vi "更新update.vi"() -> ()   [LabVIEW 2016, in "自动更新.lvlib"]
uses:
  <vilib>/FTP/NI_FTP.lvlib
panel:
  out "本地路径":path
  out "FTP链接结束":bool
  out "更新进度":u8(slide) scale=0.0..100.0
  # "更新update，请稍后！"
  # "s"
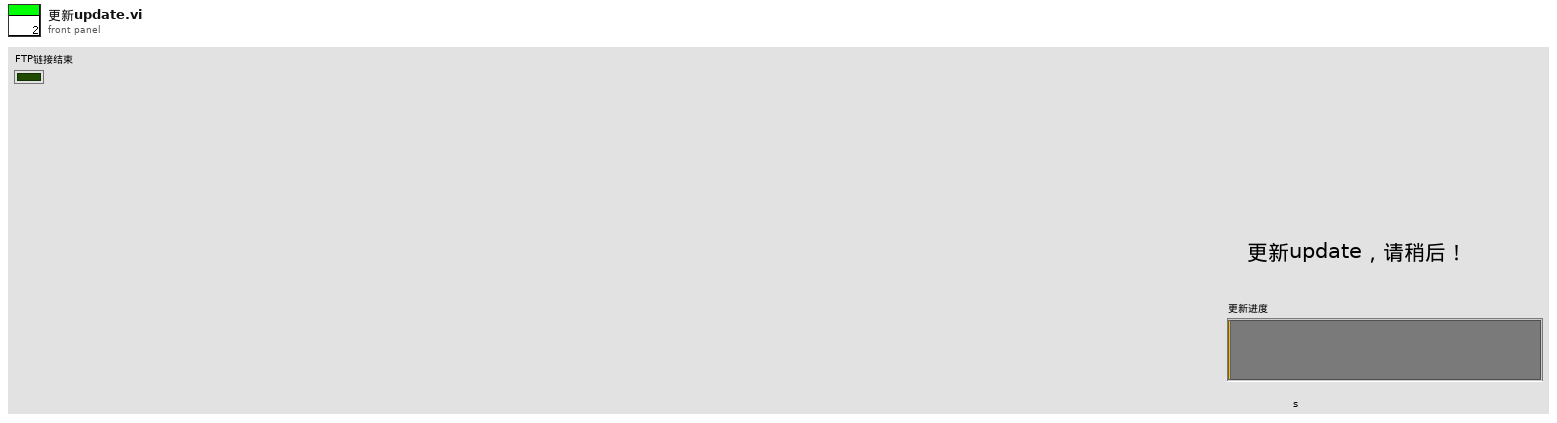
[diagram p1: front panel]
types:
  T1 = enum16{"get version information", "get success", "contact", "over"}
  T2 = cluster{"网络灯":bool, "接收中":bool, "已接收百分比":u8, "接收成功次数":dbl, "当前步骤":enum16{"init", "receivehead", "receivecontent", "receivesuccess", "over"}, "文件名":string, "error out":errorcluster}
  T3 = cluster{"remote path":string, "local path":path, "binary":bool}
  T4 = cluster{"主机":string, "用户":string, "密码":string, "远程路径":string, "下载文件名":string, "软件版本":string}
  T5 = typedef "NI_FTP.lvlib/FTP Session.ctl" = refnum<k5>
  T6 = typedef "NI_FTP.lvlib/FTP File Info.ctl" = cluster{"type":enum16{"unknown", "file", "dir", "link"}, "permissions":string, "owner":string, "group":string, "size":i32, "date":string, "name":string, "link name":string}
  T7 = cluster{"remote path":string, "local path":path, "binary":bool}[]
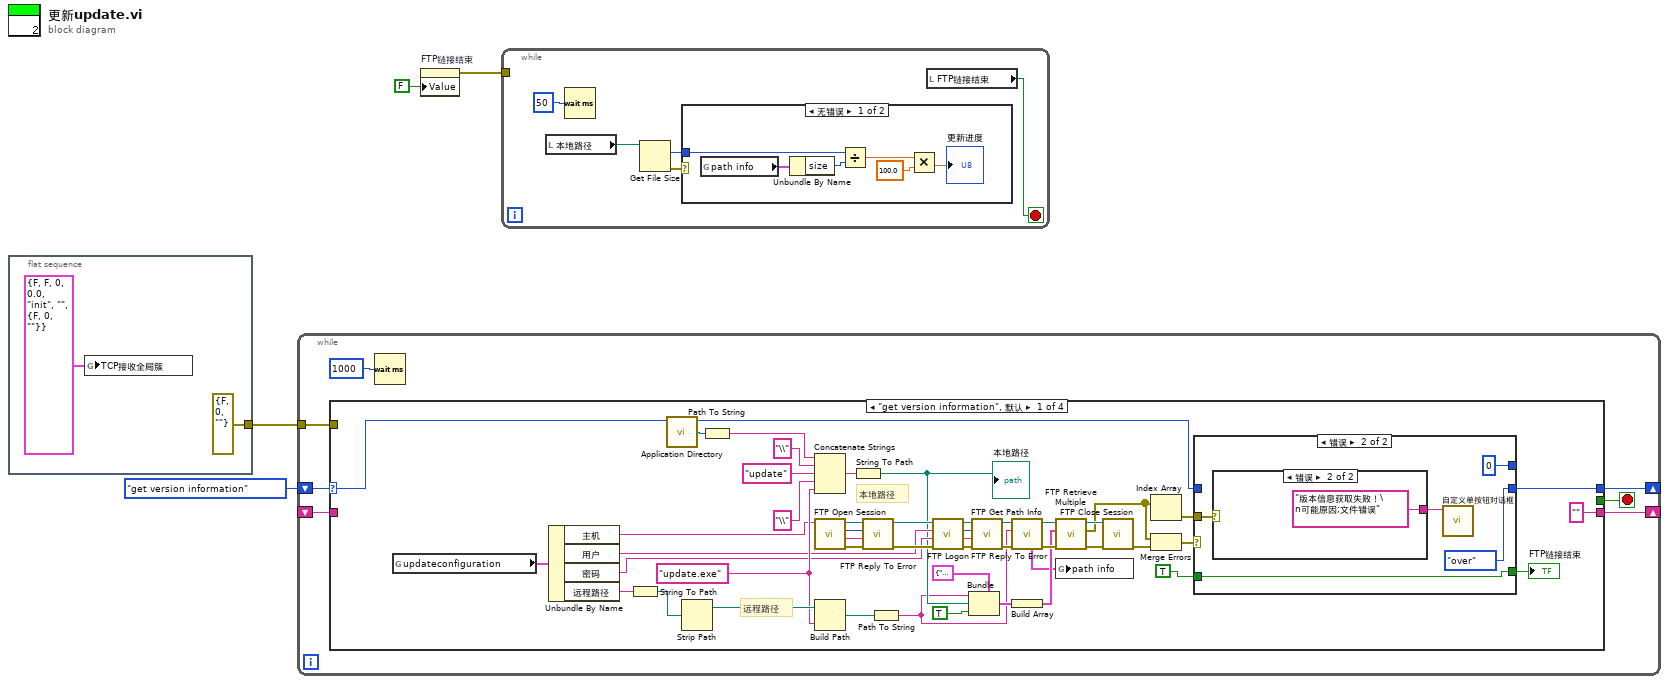
[diagram p0: block diagram]
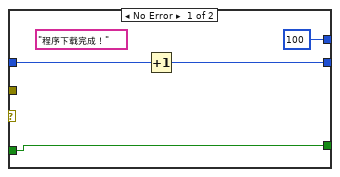
[diagram p3: hidden frame]
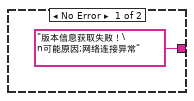
[diagram p4: hidden frame]
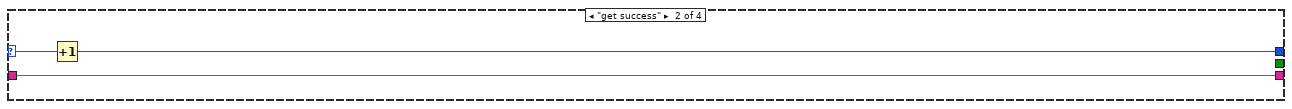
[diagram p5: hidden frame]
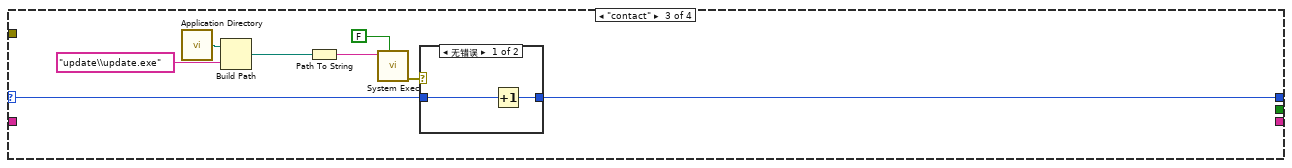
[diagram p6: hidden frame]
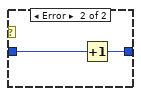
[diagram p7: hidden frame]
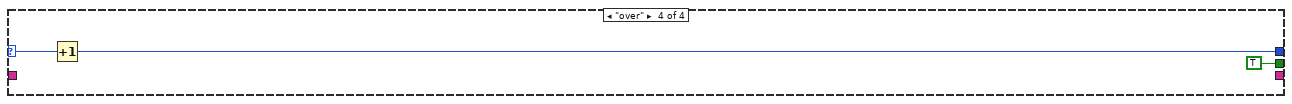
[diagram p8: hidden frame]
diagram:
  n1 = flat-sequence {
    tunnel: [errorcluster {"status"=FALSE, "code"=0, "source"=""} ("错误常量")] -> w3
    frame #0 {
      n2 = global write "全局变量1.vi" "TCP接收全局簇"(T2 {"网络灯"=FALSE, "接收中"=FALSE, "已接收百分比"=0, "接收成功次数"=0.0, "当前步骤"=enum."init", "文件名"="", "error out"={"status"=FALSE, "code"=0, "source"=""}} ("TCP接收全局簇")) -> ()
    }
  }
  n3 = while {
    shift-right: [w11] -> _
    shift-left: T1."get version information" -> [w12]
    tunnel: w3 -> [w10]
    shift-right: [w9] -> _
    shift-left: _ -> [w8]
    stop <- w7 stop-if-true
    n4 = case shown="\"get version information\", 默认" w12 {
      selector: w12 -> [w52 w74 w76 w88]
      tunnel: [w53 w73 w82 w87] -> w11
      tunnel: w10 -> [_ _ _ _]
      tunnel: ["" w72 _ _] -> w9
      tunnel: w8 -> [_ w72 _ _]
      tunnel: [_ _ _ TRUE] -> w7
      frame "get version information", Default {
        w46 = "update.exe" ("字符串")
        # "本地路径"
        # "远程路径"
        n5 = global read "update全局.vi" "updateconfiguration"() -> (w51:T4)
        n6 = Unbundle By Name(w51) -> ("主机"=w20:string, "用户"=w21:string, "密码"=w22:string, "远程路径"=w23:string)
        n7 = String To Path(string=w23) -> (path=w50:path)
        n8 = call <vilib>:"Application Directory.vi"() -> ("Application Directory"=w56:path)
        n9 = Strip Path(path=w50) -> (stripped path=w49:path)  [unwired: 1 out]
        n10 = Path To String(path=w56) -> (string=w59:string)
        n11 = Concatenate Strings(w59, "\\" ("字符串"), "update" ("字符串"), "\\" ("字符串"), w46) -> (w55:string)
        n12 = call <vilib>:"FTP Open Session.vi"("address"=w20) -> ("error out"=w35:errorcluster, "reply string"=w37:string, "reply code"=w36:i32, "ftp session"=w34:T5)  [unwired: 3 in, 4 out]
        n13 = Build Path(base path=w49, name or relative path=w46) -> (appended path=w48:path)
        n14 = String To Path(string=w55) -> (path=w19:path)
        "本地路径" <- w19
        n15 = call <vilib>:"FTP Reply To Error.vi"("error in (no error)"=w35, "reply string in"=w37, "reply code in"=w36, "ftp session"=w34) -> ("error out"=w38:errorcluster, "ftp session out"=w39:T5)  [unwired: 2 out]
        n16 = Path To String(path=w48) -> (string=w18:string)
        n17 = call <vilib>:"FTP Logon.vi"("error in (no error)"=w38, "password"=w22, "user"=w21, "ftp session"=w39) -> ("error out"=w40:errorcluster, "reply string"=w42:string, "reply code"=w43:i32, "ftp session out"=w41:T5)  [unwired: 4 out]
        n18 = Bundle(cluster=T3 {"remote path"="", "local path"=path "", "binary"=FALSE} ("transfer spec"), "remote path"=w18, "local path"=w19, "binary"=TRUE) -> (w33:T3)
        n19 = call <vilib>:"FTP Reply To Error.vi"("error in (no error)"=w40, "reply string in"=w42, "reply code in"=w43, "ftp session"=w41) -> ("error out"=w45:errorcluster, "ftp session out"=w44:T5)  [unwired: 2 out]
        n20 = call <vilib>:"FTP Get Path Info.vi"("error in (no error)"=w45, "remote path"=w18, "ftp session"=w44) -> ("error out"=w29:errorcluster, "ftp session out"=w30:T5, "path info"=w24:T6)  [unwired: 4 in, 2 out]
        n21 = Build Array(w33) -> (w28:T7)
        n22 = call <vilib>:"FTP Retrieve Multiple.vi"("error in (no error)"=w29, "file specifications"=w28, "ftp session"=w30) -> ("error out"=w26:errorcluster, "file errors"=w17:errorcluster[], "ftp session out"=w27:T5)  [unwired: 2 in, 4 out]
        n23 = global write "update全局.vi" "path info"(w24) -> ()
        n24 = call <vilib>:"FTP Close Session.vi"("error in (no error)"=w26, "ftp session"=w27) -> ("error out"=w25:errorcluster)  [unwired: 9 out]
        n25 = Index Array(array=w17) -> (element=w16:errorcluster)  [unwired: 1 in]
        n26 = Merge Errors(w17, w25) -> (w54:errorcluster)
        n27 = case shown="错误" w54 {
          tunnel: w16 -> [_ w68]
          tunnel: [u8 100 ("y") u8 0 ("y")] -> _
          tunnel: [w63 T1."over"] -> w53
          tunnel: w52 -> [w62 _]
          tunnel: [w61 w65] -> w15
          tunnel: TRUE -> [w61 w65]
          frame No Error {
            (unwired) "程序下载完成！"
            n28 = Increment(x=w62) -> (x+1=w63:T1)
          }
          frame Error {
            n29 = case shown="错误" w68 {
              tunnel: ["版本信息获取失败！\n可能原因;网络连接异常" "版本信息获取失败！\n可能原因;文件错误"] -> w69
              frame No Error {
              }
              frame Error {
              }
            }
            n30 = call "自定义单按钮对话框.vi"("消息"=w69) -> ()  [unwired: 11 in]
          }
        }
        "FTP链接结束" <- w15
      }
      frame "get success" {
        n31 = Increment(x=w74) -> (x+1=w73:T1)
      }
      frame "contact" {
        n32 = call <vilib>:"Application Directory.vi"() -> ("Application Directory"=w79:path)
        n33 = Build Path(base path=w79, name or relative path="update\\update.exe" ("字符串")) -> (appended path=w80:path)
        n34 = Path To String(path=w80) -> (string=w77:string)
        n35 = call <vilib>:"System Exec.vi"("wait until completion? (T)"=FALSE, "command line"=w77) -> ("error out"=w75:errorcluster)  [unwired: 6 in, 3 out]
        n36 = case shown="无错误" w75 {
          tunnel: w76 -> [w84 w86]
          tunnel: [w83 w85] -> w82
          frame No Error {
            n37 = Increment(x=w84) -> (x+1=w83:T1)
          }
          frame Error {
            n38 = Increment(x=w86) -> (x+1=w85:T1)
          }
        }
      }
      frame "over" {
        n39 = Increment(x=w88) -> (x+1=w87:T1)
      }
    }
    n40 = Wait (ms)(milliseconds to wait=u32 1000 ("等待时间（毫秒）")) -> ()  [unwired: 1 out]
  }
  n41 = property on="FTP链接结束" class="Bool (严格)"("Value"=FALSE ("FTP链接结束")) -> (error out=w1:errorcluster)  [unwired: 2 in, 1 out]
  n42 = while {
    tunnel: w1 -> [_]
    stop <- w94 stop-if-true
    n43 = local read "本地路径"() -> (w92:path)
    n44 = Wait (ms)(milliseconds to wait=u32 50 ("等待时间（毫秒）")) -> ()  [unwired: 1 out]
    n45 = Get File Size(file=w92) -> (size (in bytes)=w90:i64, 0:w91:errorcluster)  [unwired: 1 in, 1 out]
    n46 = case shown="无错误" w91 {
      tunnel: w90 -> [w96 _]
      frame No Error {
        n47 = global read "update全局.vi" "path info"() -> (w97:T6)
        n48 = Unbundle By Name(w97) -> ("size"=w100:i32)
        n49 = Divide(x=w96, y=w100) -> (x/y=w99:dbl)
        n50 = Multiply(x=w99, y=100.0) -> (x*y=→"更新进度":dbl)
      }
      frame Error {
      }
    }
    n51 = local read "FTP链接结束"() -> (w94:bool)
  }
